vi "zipToJson.vi"(4 "passYield":dbl, 5 "DBSet":T1, 6 "uploadPath":path, 7 "successxmlpath":path, 8 "转换失败路径":path, 9 "目标路径":path, 10 "status msg ref":refnum<vi>, 11 "path":path caption="zip path") -> ()   [LabVIEW 2011]
panel:
  out "customerPN":string
  out "usedSN":string
  out "result":string
  out "upload":bool
  out "archive name out":path
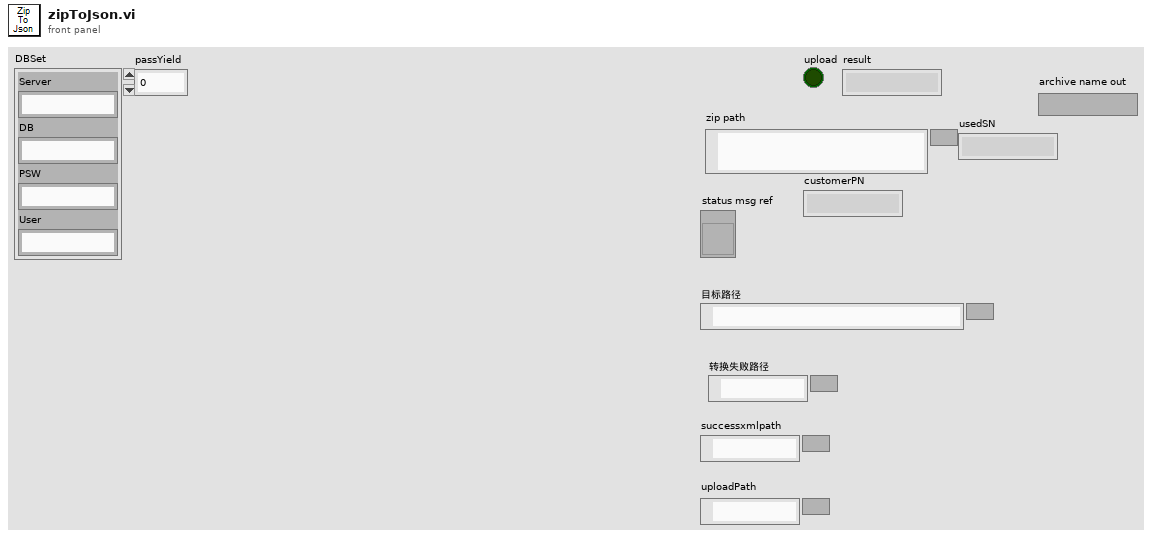
[diagram p1: front panel]
types:
  T1 = cluster{"Server":string, "DB":string, "PSW":string, "User":string}
  T2 = typedef "TDD.ctl" = cluster{"show_Cable Point":dbl[], "show_Terminal Point":dbl[], "show_impspec":string[]}
  T3 = typedef "xml_detail.ctl" = cluster{"FileVersion":string, "FileName":string, "customerPN":string, "usedSN":string, "test time":string[], "testResult":bool}
  T4 = typedef "sSpec.ctl" = cluster{"itemName":string, "upperLimit":dbl[], "lowerLimit":dbl[], "testResult":string, "result":bool}
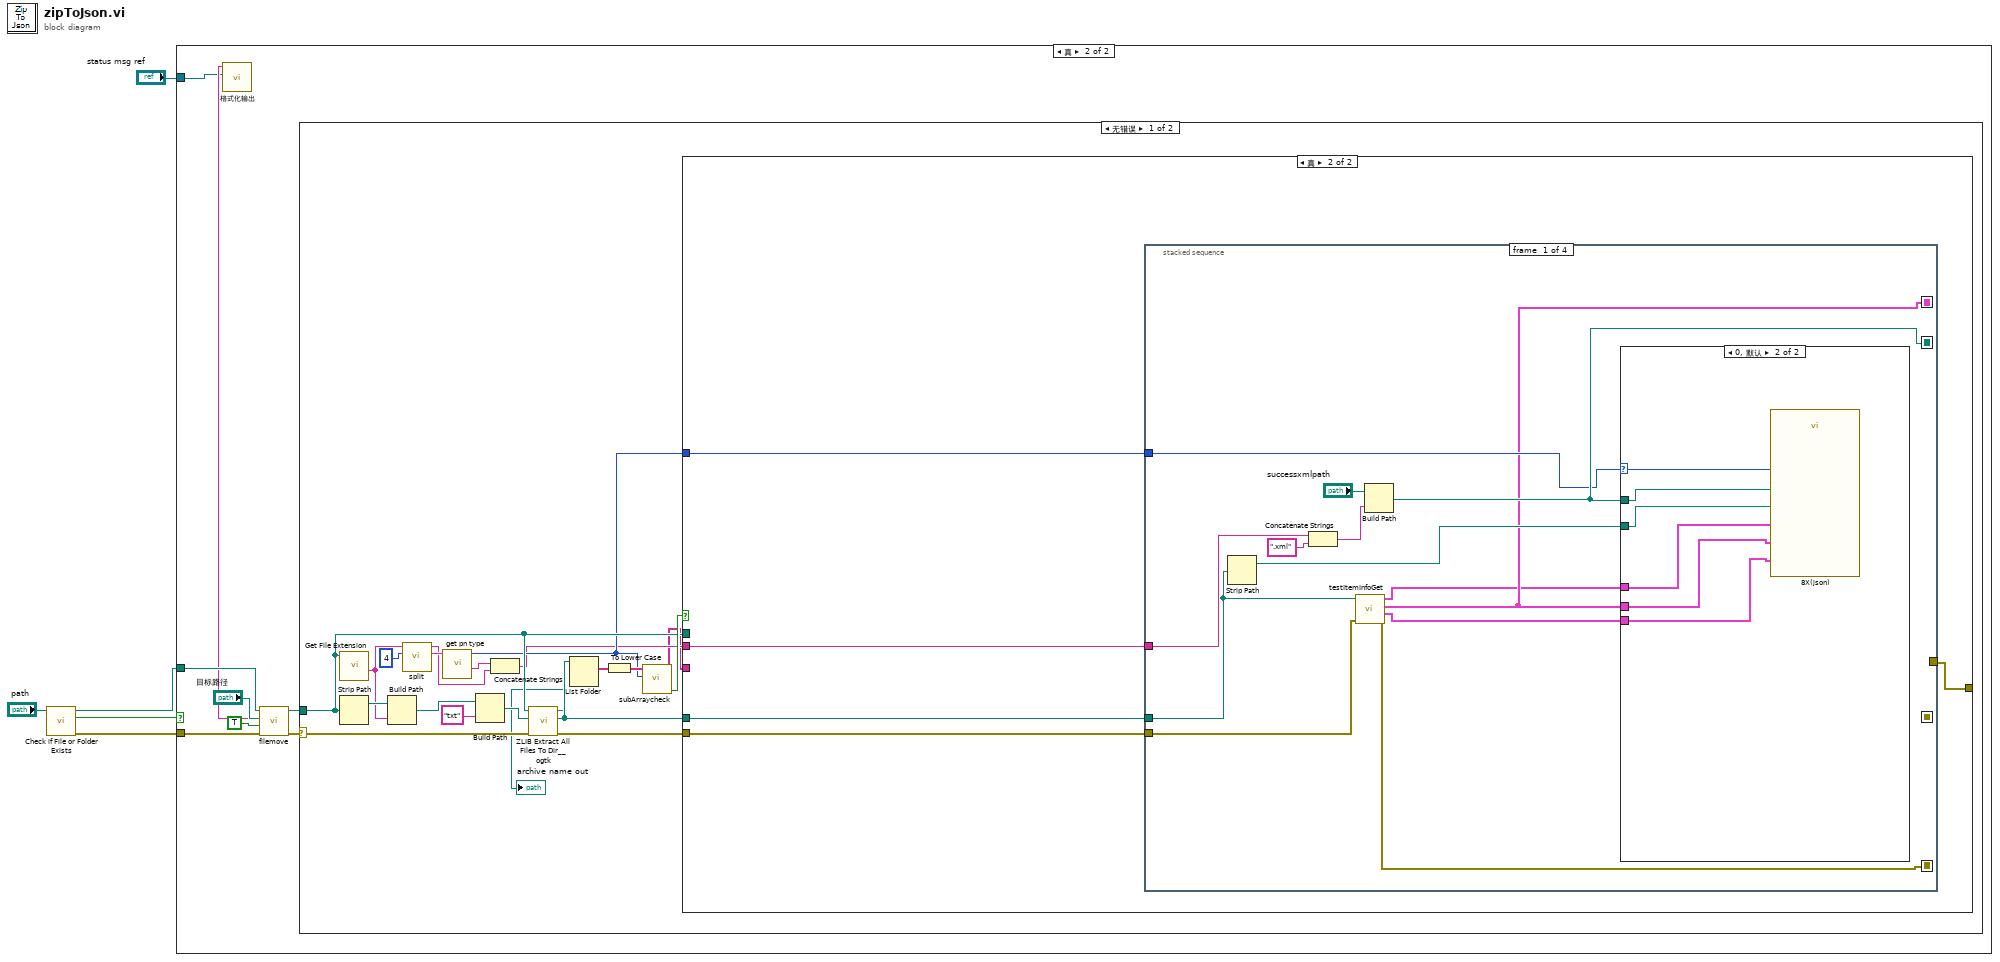
[diagram p0: block diagram]
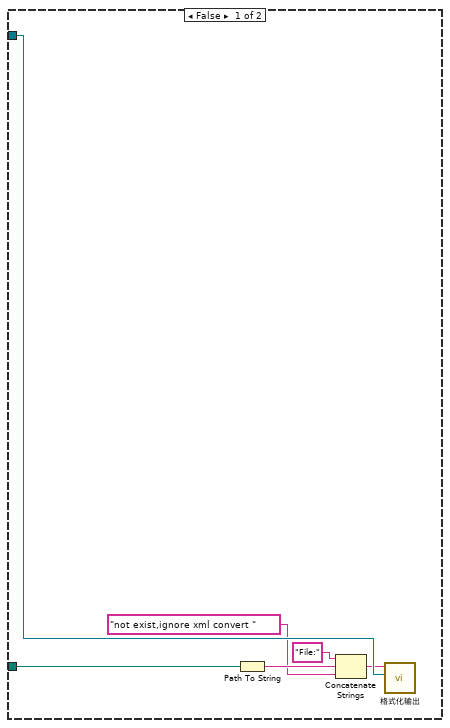
[diagram p2: hidden frame]
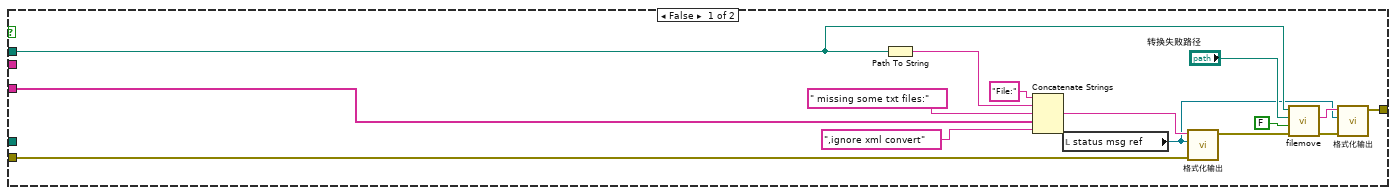
[diagram p3: hidden frame]
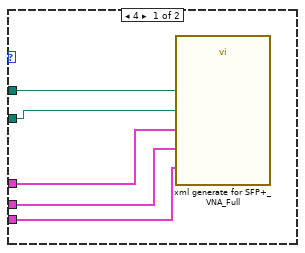
[diagram p4: hidden frame]
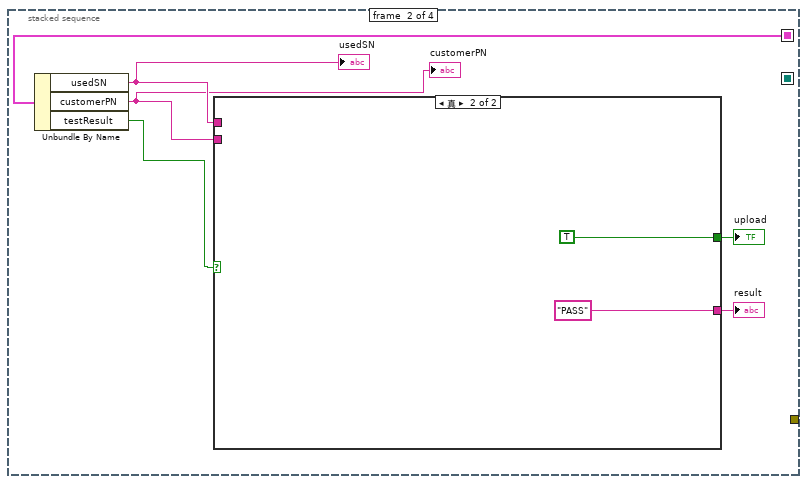
[diagram p5: hidden frame]
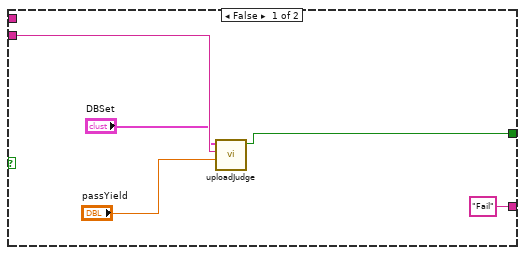
[diagram p6: hidden frame]
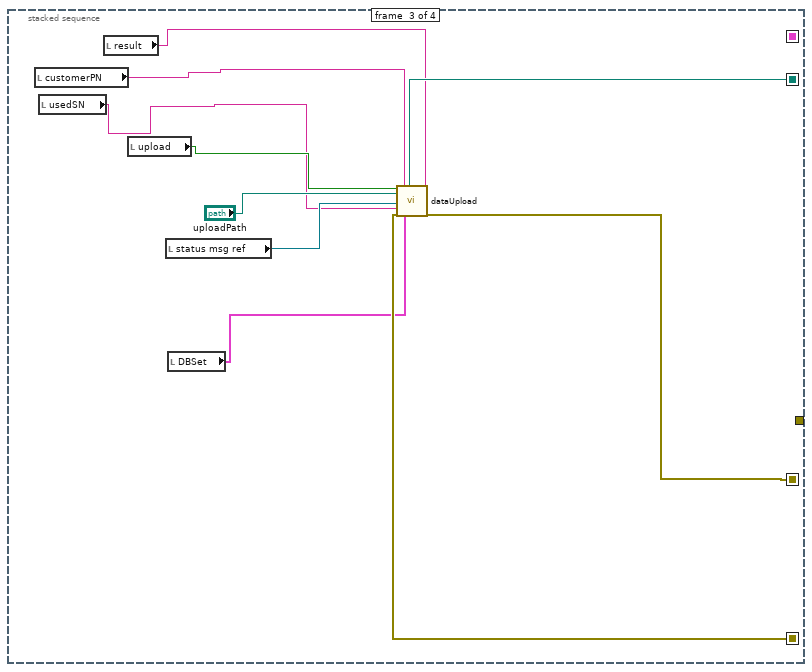
[diagram p7: hidden frame]
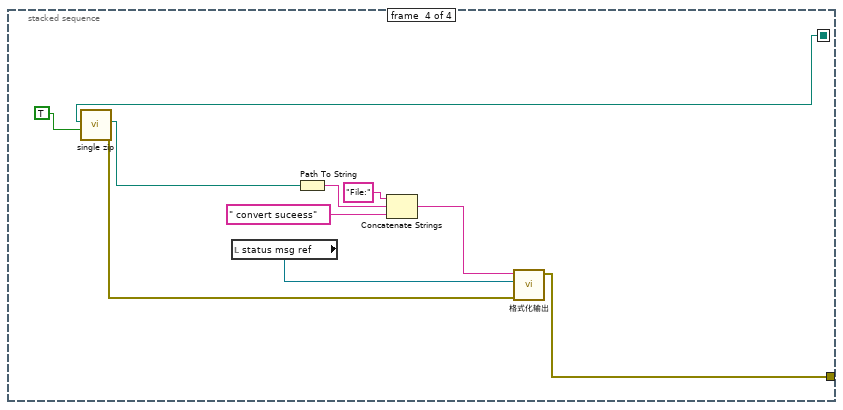
[diagram p8: hidden frame]
diagram:
  n1 = call <vilib>:"Check if File or Folder Exists.vi"("path"="path") -> ("error out"=w2:errorcluster, "file or folder exists?"=w5:bool, "dup path"=w4:path)  [unwired: 8 in]
  n2 = case shown="真" w5 {
    tunnel: w4 -> [w10 w19]
    tunnel: "status msg ref" -> [w11 w14]
    tunnel: w2 -> [_ w12]
    frame False {
      n3 = Path To String(path=w10) -> (string=w8:string)
      n4 = Concatenate Strings("File:" ("字符串"), w8, "not exist,ignore xml convert " ("字符串")) -> (w6:string)
      n5 = call "格式化输出.vi"("字符串引用"=w11, "字符串"=w6) -> ()  [unwired: 9 in, 1 out]
    }
    frame True {
      n6 = call "filemove.vi"("错误输入"=w12, "清空"=TRUE, "目标路径"="目标路径", "源路径"=w19) -> ("错误输出"=w18:errorcluster, "msg"=w15:string, "新路径"=w17:path)  [unwired: 5 in]
      n7 = call "格式化输出.vi"("字符串引用"=w14, "字符串"=w15) -> ()  [unwired: 9 in, 1 out]
      n8 = case shown="无错误" w18 {
        selector: w18 -> [w31 _]
        tunnel: w17 -> [w32 _]
        frame No Error {
          n9 = call <nishared>:"Get File Extension.vi"("file"=w32) -> ("filename without extension"=w28:string)  [unwired: 7 in, 3 out]
          n10 = Strip Path(path=w32) -> (stripped path=w39:path)  [unwired: 1 out]
          n11 = Build Path(base path=w39, name or relative path=w28) -> (appended path=w38:path)
          n12 = call "split.vi"("长度"=4, "source"=w28) -> ("left"=w26:string, "right"=w21:string)  [unwired: 8 in]
          n13 = call "get pn type.vi"("字符串"=w26) -> ("type adder"=w22:string, "type"=w25:i32)  [unwired: 9 in]
          n14 = Build Path(base path=w38, name or relative path="txt" ("名称或相对路径")) -> (appended path=w36:path)
          n15 = Concatenate Strings(w22, w21) -> (w23:string)
          n16 = call <userlib>:"ZLIB Extract All Files To Dir__ogtk.vi"("error in (no error)"=w31, "root directory (archive name without ending)"=w36, "archive name (file dialog)"=w32) -> ("error out"=w30:errorcluster, "root directory out"=w35:path, "archive name out"=→"archive name out":path)  [unwired: 6 in]
          n17 = List Folder(path=w35) -> (filenames=w29:string[])  [unwired: 3 in, 3 out]
          n18 = To Lower Case(string=w29) -> (all lower case string=w34:string[])
          n19 = call "subArraycheck.vi"("type"=w25, "source"=w34) -> ("is in?"=w33:bool, "diff element"=w20:string[])  [unwired: 8 in]
          n20 = case shown="真" w33 {
            tunnel: w23 -> [_ w59]
            tunnel: w35 -> [_ w58]
            tunnel: w32 -> [w52 _]
            tunnel: w30 -> [w43 w57]
            tunnel: [w42 w55] -> _
            tunnel: w25 -> [_ w56]
            tunnel: w20 -> [w41 _]
            frame False {
              n21 = Path To String(path=w52) -> (string=w50:string)
              n22 = Concatenate Strings("File:" ("字符串"), w50, " missing some txt files:" ("字符串"), w41, ",ignore xml convert") -> (w48:string)
              n23 = local read "status msg ref"() -> (w46:refnum<vi>)
              n24 = call "格式化输出.vi"("错误输入（无错误）"=w43, "字符串引用"=w46, "字符串"=w48) -> ("错误输出"=w45:errorcluster)  [unwired: 8 in]
              n25 = call "filemove.vi"("错误输入"=w45, "清空"=FALSE, "目标路径"="转换失败路径", "源路径"=w52) -> ("错误输出"=w44:errorcluster, "msg"=w47:string)  [unwired: 5 in, 1 out]
              n26 = call "格式化输出.vi"("错误输入（无错误）"=w44, "字符串引用"=w46, "字符串"=w47) -> ("错误输出"=w42:errorcluster)  [unwired: 8 in]
            }
            frame True {
              n27 = stacked-sequence {
                seq-local: [w68 _ _ _] -> [_ _ w102 w116]
                seq-local: [w60 _ _ _] -> [_ _ w105 _]
                seq-local: [_ _ w104 _] -> [_ _ _ _]
                seq-local: [w64 _ _ _] -> [_ w85 _ _]
                tunnel: w59 -> [w71 _ _ _]
                tunnel: w58 -> [w65 _ _ _]
                tunnel: w57 -> [w61 _ _ _]
                tunnel: w56 -> [w66 _ _ _]
                tunnel: [_ _ _ w107] -> w55
                frame #0 {
                  n28 = Strip Path(path=w65) -> (stripped path=w72:path)  [unwired: 1 out]
                  n29 = Concatenate Strings(w71, ".xml" ("字符串")) -> (w69:string)
                  n30 = call "testItemInfoGet.vi"("error in (no error)"=w61, "basePath"=w65) -> ("error out"=w60:errorcluster, "TDD"=w62:T2, "xml_detail"=w64:T3, "singleItemInfo"=w63:T4[])  [unwired: 6 in]
                  n31 = Build Path(base path="successxmlpath", name or relative path=w69) -> (appended path=w68:path)
                  n32 = case shown="0, 默认" w66 {
                    selector: w66 -> [_ w83]
                    tunnel: w72 -> [w76 w81]
                    tunnel: w68 -> [w77 w82]
                    tunnel: w64 -> [w74 w79]
                    tunnel: w63 -> [w75 w80]
                    tunnel: w62 -> [w73 w78]
                    frame 4 {
                      n33 = call "xml generate for SFP+_VNA_Full.vi"("xmlPath"=w77, "txtPath"=w76, "singleItemInfo"=w75, "xml_detail"=w74, "TDD"=w73) -> ()  [unwired: 11 in]
                    }
                    frame 0, Default {
                      n34 = call "8X(json).vi"("xml path"=w82, "type"=w83, "txtPath"=w81, "singleItemInfo"=w80, "xml_detail"=w79, "TDD"=w78) -> ()  [unwired: 10 in]
                    }
                  }
                }
                frame #1 {
                  n35 = Unbundle By Name(w85) -> ("usedSN"=w89:string, "customerPN"=w88:string, "testResult"=w84:bool)
                  "usedSN" <- w89
                  "customerPN" <- w88
                  n36 = case shown="真" w84 {
                    tunnel: [w93 TRUE] -> w87
                    tunnel: ["Fail" "PASS"] -> w86
                    tunnel: w89 -> [_ _]
                    tunnel: w88 -> [w91 _]
                    frame False {
                      n37 = call "uploadJudge.vi"("passYield"="passYield", "pn"=w91, "DBSet"="DBSet") -> ("upload"=w93:bool)  [unwired: 8 in]
                    }
                    frame True {
                    }
                  }
                  "upload" <- w87
                  "result" <- w86
                }
                frame #2 {
                  n38 = local read "customerPN"() -> (w99:string)
                  n39 = local read "usedSN"() -> (w98:string)
                  n40 = local read "result"() -> (w100:string)
                  n41 = local read "upload"() -> (w101:bool)
                  n42 = local read "status msg ref"() -> (w103:refnum<vi>)
                  n43 = local read "DBSet"() -> (w97:T1)
                  n44 = call "dataUpload.vi"("upload"=w101, "uploadpath"="uploadPath", "status msg ref"=w103, "sn"=w98, "错误输入（无错误）"=w105, "pn"=w99, "DBSet"=w97, "xmlPath"=w102, "result"=w100) -> ("错误输出"=w104:errorcluster)  [unwired: 10 in]
                }
                frame #3 {
                  n45 = call "single zip.vi"("del source?"=TRUE, "source file path"=w116) -> ("error out"=w108:errorcluster, "output zip"=w110:path)  [unwired: 8 in]
                  n46 = local read "status msg ref"() -> (w109:refnum<vi>)
                  n47 = Path To String(path=w110) -> (string=w113:string)
                  n48 = Concatenate Strings("File:" ("字符串"), w113, " convert suceess" ("字符串")) -> (w111:string)
                  n49 = call "格式化输出.vi"("错误输入（无错误）"=w108, "字符串引用"=w109, "字符串"=w111) -> ("错误输出"=w107:errorcluster)  [unwired: 8 in]
                }
              }
            }
          }
        }
        frame Error {
        }
      }
    }
  }
